vi "Red PLC InReg.vi"(8 "error in (no error)":errorcluster, 9 "length":i32=10, 10 "index":i32, 11 "Input Registers Arr":u16[](array[numeric])=[0, 0, 0, 0, 0, 0, 0, 0]) -> (0 "error out":errorcluster, 3 "Rad In Reg":string)   [LabVIEW 2019]
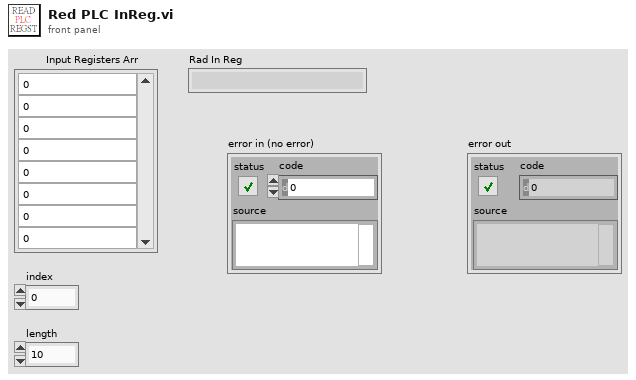
[diagram p1: front panel]
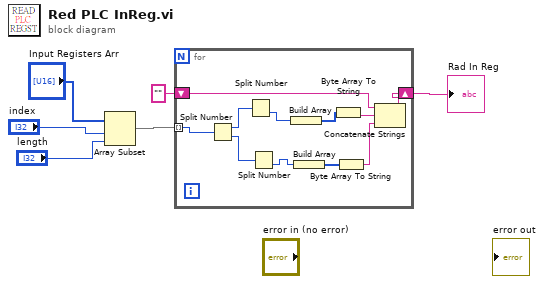
[diagram p0: block diagram]
diagram:
  n1 = Array Subset(array="Input Registers Arr", index="index", length="length") -> (w5:u16[])
  n2 = for {
    shift-right: [w10] -> w2
    shift-left: "" -> [w11]
    tunnel: w5 -> [w7] mode=indexing
    n3 = Split Number(x=w7) -> (hi(x)=w16:u8, lo(x)=w14:u8)
    n4 = Split Number(x=w16) -> (lo(x)=w9:u8)  [unwired: 1 out]
    n5 = Split Number(x=w14) -> (lo(x)=w8:u8)  [unwired: 1 out]
    n6 = Build Array(w9) -> (w17:u8[])
    n7 = Build Array(w8) -> (w15:u8[])
    n8 = Byte Array To String(unsigned byte array=w17) -> (string=w13:string)
    n9 = Byte Array To String(unsigned byte array=w15) -> (string=w12:string)
    n10 = Concatenate Strings(w11, w13, w12) -> (w10:string)
  }
  "Rad In Reg" <- w2
